vi "ProperEyeMovement.vi"(7 "State":T1, 8 "error in (no error)":errorcluster, 9 "y":dbl, 10 "x":dbl, 11 "TwoAfcEye in":refnum<class "TwoAfcEye.lvclass">) -> (0 "error out":errorcluster, 2 "CorrectEye":bool, 3 "TwoAfcEye out":refnum<class "TwoAfcEye.lvclass">)   [LabVIEW 2011, in "TwoAfcEye.lvclass"]
uses:
  TwoAfcEye.lvclass
  Trial Based Experiment Statechart/Trial Based Experiment.lvsc/State.ctl
  TwoAfcEye.lvclass/TwoAfcEye.ctl
  <vilib>/imath/engines/lvmath2/RunTimeEngine/ErrorHandling/NIMS_Finalize Error.vi
  <vilib>/imath/engines/lvmath2/RunTimeEngine/NodeEndStatement/NIMS_NodeEndStatement_Output.vi
  <instcachedir>/0/NIMS_NodeEndStatement_Output_53EC0D466D134D7ABD903AC30B43404B.lvgen/NIMS_NodeEndStatement_Output_53EC0D466D134D7ABD903AC30B43404B_009.vi
  <vilib>/imath/engines/lvmath2/RunTimeEngine/BuiltInFunctions/sum/NIMS_sum(GV).vi
  <instcachedir>/0/NIMS_sum(GV)_67F5EC36BC034E54A6BEC5B0673C00E5.lvgen/NIMS_sum(GV)_67F5EC36BC034E54A6BEC5B0673C00E5_000.vi
  <vilib>/imath/engines/lvmath2/RunTimeEngine/ArithmeticOperatorToken/NIMS_ArithmeticOperator_multmx(RV,CV)-internal.vi
  <instcachedir>/0/NIMS_ArithmeticOperator_multmx(RV,CV)-internal_26C0DCAD7F024225968CB0639EC17D76.lvgen/NIMS_ArithmeticOperator_multmx(RV,CV)-internal_26C0DCAD7F024225968CB0639EC17D76_006.vi
  <vilib>/imath/engines/lvmath2/RunTimeEngine/BuiltInFunctions/abs/NIMS_abs(signed).vi
  <instcachedir>/0/NIMS_abs(signed)_C4FCB8E6058B49B797C7C8D53CA5F6EC.lvgen/NIMS_abs(signed)_C4FCB8E6058B49B797C7C8D53CA5F6EC_002.vi
  <vilib>/imathl/engines/lvmath/Functions/Error Handling/Create Error.vi
  Trial Based Experiment Statechart/Trial Based Experiment.lvsc
panel:
  in  "incTargRad":dbl=100.0
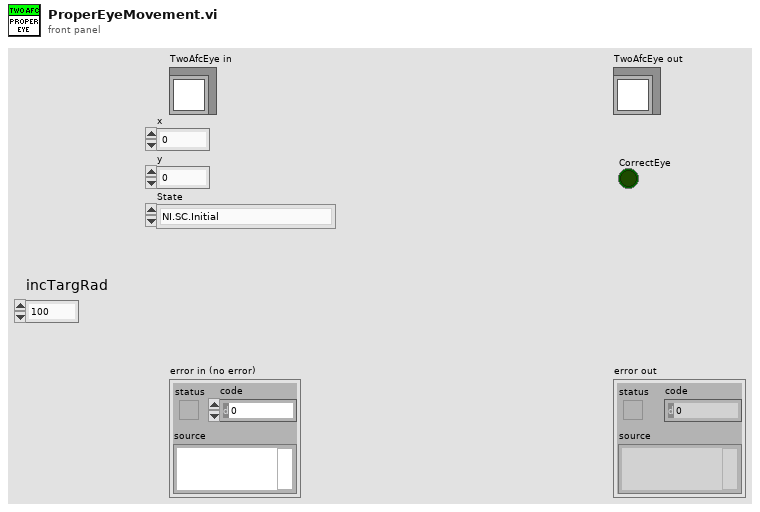
[diagram p1: front panel]
types:
  T1 = typedef "Trial Based Experiment.lvsc/State.ctl" = enum16{"NI.SC.Initial", "NI.SC.History", "NI.SC.ShallowHistory", "NI.SC.Terminal", "Cleanup", "State", "State\\Region\\Pause", "State\\Region\\Response Period", "State\\Region\\Delay Period", "State\\Region\\Hold Fixation", "State\\Region\\Acquire Fixation", "State\\Region\\Abort Trial", "State\\Region\\End Trial", "State\\Region\\Intertrial", "State\\Region\\Start Trial"}
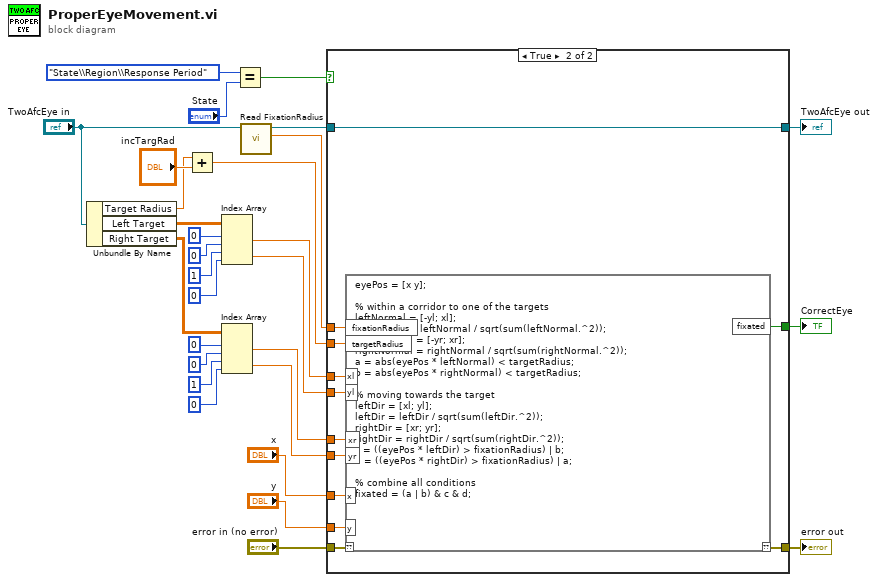
[diagram p0: block diagram]
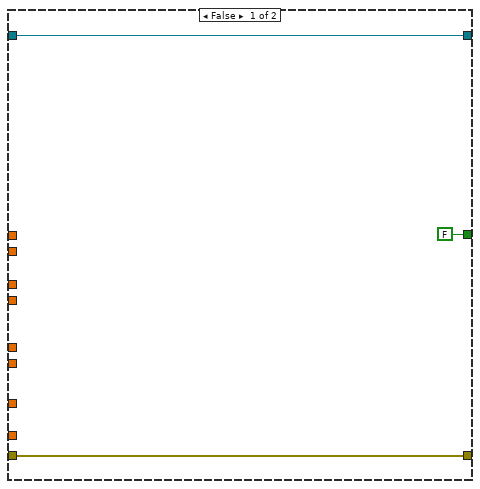
[diagram p2: hidden frame]
diagram:
  n1 = Unbundle By Name("TwoAfcEye in") -> ("Target Radius"=w5:dbl, "Left Target"=w4:dbl[][], "Right Target"=w3:dbl[][])
  n2 = Add(x=w5, y="incTargRad") -> (x+y=w17:dbl)
  n3 = Index Array(array=w4, index (row) #1=0 ("index"), index (col) #1=0 ("disabled index (col)"), index (row) #2=1 ("index"), index (col) #2=0 ("disabled index (col)")) -> (element #1=w21:dbl, element #2=w20:dbl)
  n4 = Index Array(array=w3, index (row) #1=0 ("index"), index (col) #1=0 ("disabled index (col)"), index (row) #2=1 ("index"), index (col) #2=0 ("disabled index (col)")) -> (element #1=w19:dbl, element #2=w18:dbl)
  n5 = Equal?(x=State."State\\Region\\Response Period", y="State") -> (x = y?=w9:bool)
  n6 = call-dynamic "Read FixationRadius.vi"("MatlabExperiment in"="TwoAfcEye in") -> ("FixationRadius"=w7:dbl, "MatlabExperiment out"=w2:refnum<class "TwoAfcEye.lvclass">)  [unwired: 8 in, 1 out]
  n7 = case shown="True" w9 {
    tunnel: w21 -> [_ w44]
    tunnel: w20 -> [_ w43]
    tunnel: w19 -> [_ w42]
    tunnel: w18 -> [_ w41]
    tunnel: w7 -> [_ w40]
    tunnel: [FALSE ("fixated") w39] -> w8
    tunnel: w17 -> [_ w38]
    tunnel: "x" -> [_ w37]
    tunnel: "y" -> [_ w36]
    tunnel: "error in (no error)" -> [w30 w35]
    tunnel: [w30 w34] -> w12
    tunnel: w2 -> [w31 w33]
    tunnel: [w31 w33] -> w1
    frame False {
    }
    frame True {
      n8 = mathscript code="eyePos = [x y];\n\n% within a corridor to one of the targets\nleftNormal = [-yl; xl];\nleftNormal = leftNormal / sqrt(sum(leftNormal.^2));\nrightNormal = [-yr; xr];\nrightNormal = rightNormal / sqrt(sum(rightNormal.^2));\na = abs(eyePos * leftNormal) < targetRadius;\nb = abs(eyePos * rightNormal) < targetRadius;\n\n% moving towards the target\nleftDir = [xl; yl];\nleftDir = leftDir / sqrt(sum(leftDir.^2));\nrightDir = [xr; yr];\nrightDir = rightDir / sqrt(sum(rightDir.^2));\nc = ((eyePos * leftDir) > fixationRadius) | b;\nd = ((eyePos * rightDir) > fixationRadius) | a;\n\n% combine all conditions\nfixated = (a | b) & c & d;"("??"=w35, "xl"=w44, "yl"=w43, "xr"=w42, "yr"=w41, "fixationRadius"=w40, "targetRadius"=w38, "x"=w37, "y"=w36) -> ("??"=w34:errorcluster, "fixated"=w39:bool)
    }
  }
  "error out" <- w12
  "TwoAfcEye out" <- w1
  "CorrectEye" <- w8
